vi "Initialize UDP.vi"(8 "error in":errorcluster, 11 "Telnet V2 in":refnum<class "Telnet V2.lvclass">) -> (0 "error out":errorcluster, 3 "connection ID":refnum<k16>)   [LabVIEW 2018, in "Telnet V2.lvlib" / "Telnet V2.lvclass"]
uses:
  Telnet V2.lvclass
  C:/AME Test Engineering/LabVIEW/PPLs/LiDAR/Parent/LiDAR.lvlibp/LiDAR.lvclass
  PPLs/Configuration/Configuration.lvlibp/Configuration.lvclass
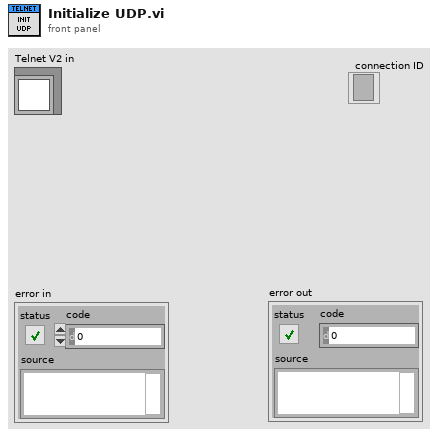
[diagram p1: front panel]
types:
  T1 = cluster{"Configuration":refnum<class "Configuration.lvclass">, "Network":cluster{"TCP":cluster{"IP Address":string, "Port":u16}, "UDP":cluster{"IP Address":string, "Port":u16}}, "Azimuth":cluster{"Min >=-60":string, "Max <=+60":string}, "Elevation":cluster{"FOV":string, "Offset":string, "Scan Pattern":enum16{"Triangle", "Snap"}, "Frequency":string}, "Data Algo":enum16{"Resim", "Point Cloud"}}
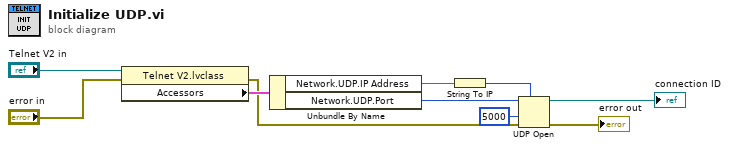
[diagram p0: block diagram]
diagram:
  n1 = property class="Telnet V2.lvclass"(reference="Telnet V2 in", error in="error in") -> (error out=w2:errorcluster, "Accessors"=w10:T1)  [unwired: 1 out]
  n2 = Unbundle By Name(w10) -> ("Network.UDP.IP Address"=w8:string, "Network.UDP.Port"=w9:u16)
  n3 = String To IP(1:w8) -> (0:w7:u32)
  n4 = UDP Open(7:w7, 8:w2, 9:5000 ("timeout ms (25000)"), 11:w9) -> (port=→"connection ID":refnum<k16>, 0:→"error out":errorcluster)  [unwired: 1 in, 1 out]
